vi "Fluke8808_Measure.vi"(8 "error in":errorcluster, 10 "Read From Display":u16(ring) items=["Primary", "Secondary ", "Both"], 11 "MyIndex":u8) -> (0 "error out":errorcluster, 1 "Secondary Display Measurement":dbl, 2 "Primary Display Measurement":dbl format="%#_6f", 3 "VISA resource":refnum<visa-resource-name>, 4 "Secondary Display Units":string, 5 "Primary Display Units":string)   [LabVIEW 2015]
doc: "Reads and returns a single measurement from the instrument."
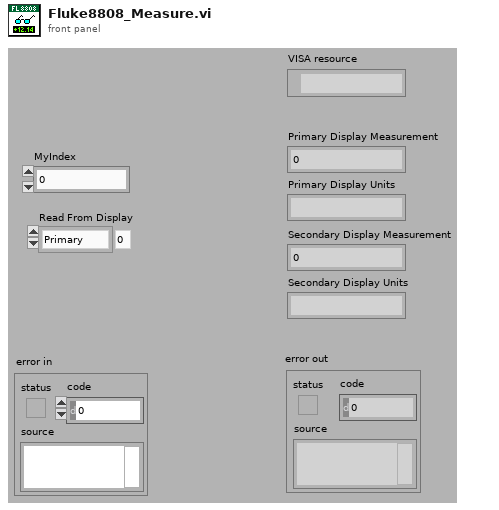
[diagram p1: front panel]
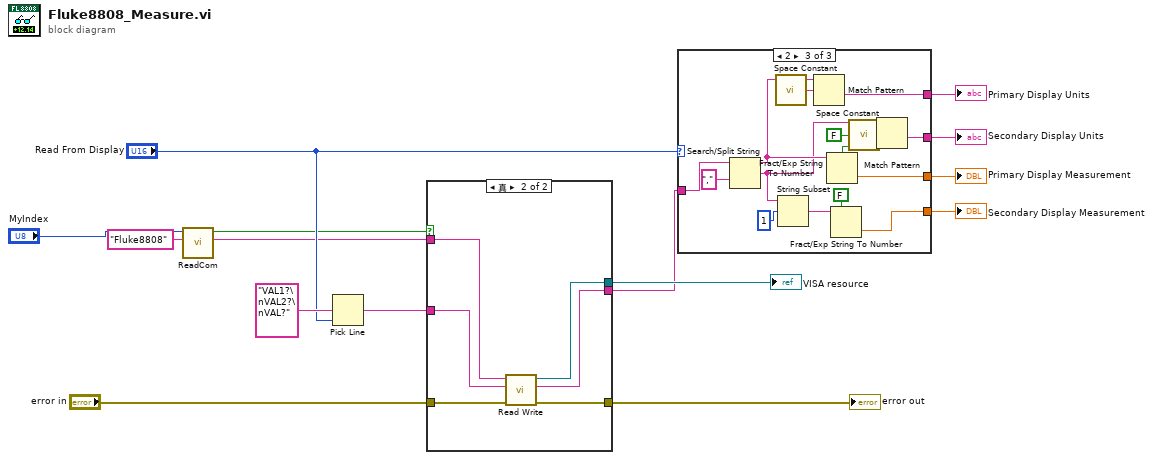
[diagram p0: block diagram]
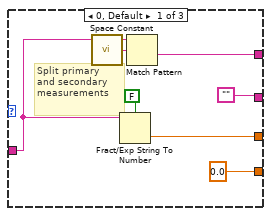
[diagram p3: hidden frame]
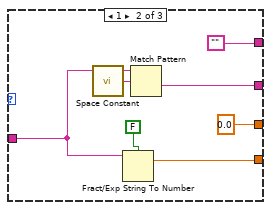
[diagram p4: hidden frame]
diagram:
  n1 = call "ReadCom.vi"("仪器名称"="Fluke8808", "MyIndex"="MyIndex") -> ("COM"=w2:string, "OK?"=w1:bool)  [unwired: 7 in, 1 out]
  n2 = Pick Line(multi-line string="VAL1?\nVAL2?\nVAL?" ("Take Measurements"), line index="Read From Display") -> (output string=w12:string)  [unwired: 1 in]
  n3 = case shown="真" w1 {
    tunnel: [_ w22] -> w15
    tunnel: [w16 w21] -> w14
    tunnel: w12 -> [_ w20]
    tunnel: [_ w19] -> w11
    tunnel: "error in" -> [w16 w18]
    tunnel: w2 -> [_ w17]
    frame False {
    }
    frame True {
      n4 = call "Read Write.vi"("error in (no error)"=w18, "Write String"=w20, "VISA resource name"=w17) -> ("error out"=w21:errorcluster, "Read Data"=w19:string, "VISA resource name out"=w22:refnum<visa-resource-name>)  [unwired: 6 in]
    }
  }
  "VISA resource" <- w15
  "error out" <- w14
  n5 = case shown="2" "Read From Display" {
    tunnel: w11 -> [w26 w34 w50]
    tunnel: [0.0 w31 w40] -> w9
    tunnel: [w24 0.0 w41] -> w8
    tunnel: [w27 "" w46] -> w7
    tunnel: ["" w32 w42] -> w6
    frame 0, Default {
      # "Split primary\nand secondary\nmeasurements"
      n6 = call <vilib>:"Space Constant.vi"() -> ("String"=w25:string)
      n7 = Fract/Exp String To Number(use system decimal point (T)=FALSE, string=w26) -> (number=w24:dbl)  [unwired: 2 in, 1 out]
      n8 = Match Pattern(string=w26, regular expression=w25) -> (after substring=w27:string)  [unwired: 1 in, 3 out]
    }
    frame 1 {
      n9 = call <vilib>:"Space Constant.vi"() -> ("String"=w35:string)
      n10 = Fract/Exp String To Number(use system decimal point (T)=FALSE, string=w34) -> (number=w31:dbl)  [unwired: 2 in, 1 out]
      n11 = Match Pattern(string=w34, regular expression=w35) -> (after substring=w32:string)  [unwired: 1 in, 3 out]
    }
    frame 2 {
      n12 = Search/Split String(string=w50, search string/char (-)=",") -> (substring before match=w45:string, match + rest of string=w43:string)  [unwired: 1 in, 1 out]
      n13 = call <vilib>:"Space Constant.vi"() -> ("String"=w44:string)
      n14 = String Subset(string=w43, offset (0)=1) -> (substring=w47:string)  [unwired: 1 in]
      n15 = Match Pattern(string=w45, regular expression=w44) -> (after substring=w46:string)  [unwired: 1 in, 3 out]
      n16 = Fract/Exp String To Number(use system decimal point (T)=FALSE, string=w45) -> (number=w41:dbl)  [unwired: 2 in, 1 out]
      n17 = Fract/Exp String To Number(use system decimal point (T)=FALSE, string=w47) -> (number=w40:dbl)  [unwired: 2 in, 1 out]
      n18 = call <vilib>:"Space Constant.vi"() -> ("String"=w39:string)
      n19 = Match Pattern(string=w43, regular expression=w39) -> (after substring=w42:string)  [unwired: 1 in, 3 out]
    }
  }
  "Secondary Display Measurement" <- w9
  "Primary Display Measurement" <- w8
  "Primary Display Units" <- w7
  "Secondary Display Units" <- w6
